vi "De-NaNArray.vi"(3 "ArrayIn":dbl[](array[numeric])) -> (0 "GoodFraction":dbl, 1 "de-NaN-dArrayOut":dbl[](array[numeric]))   [LabVIEW 2013]
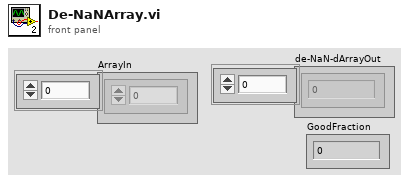
[diagram p1: front panel]
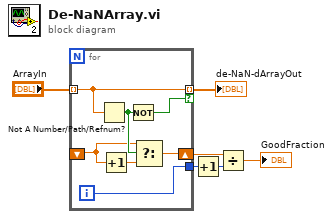
[diagram p0: block diagram]
diagram:
  n1 = for {
    tunnel: "ArrayIn" -> [w13] mode=indexing
    tunnel: [w13] -> w5 mode=indexing if=w12
    shift-right: [w11] -> w4
    shift-left: _ -> [w8]
    tunnel: [w7] -> w3
    i -> [w7]
    n2 = Not A Number/Path/Refnum?(number/path/refnum=w13) -> (NaN/Path/Refnum?=w10:bool)
    n3 = Increment(x=w8) -> (x+1=w9:dbl)
    n4 = Not(x=w10) -> (.not. x?=w12:bool)
    n5 = Select(t=w8, s=w10, f=w9) -> (s? t:f=w11:dbl)
  }
  "de-NaN-dArrayOut" <- w5
  n6 = Increment(x=w3) -> (x+1=w2:i32)
  n7 = Divide(x=w4, y=w2) -> (x/y=→"GoodFraction":dbl)
